vi "纳清pH电极校准.vi"() -> ()   [LabVIEW 2016, in "斯坦道多参数.lvlib"]
uses:
  <vilib>/Utility/miscctls.llb/LVPointTypeDef.ctl
  <vilib>/Analysis/NI_AALBase.lvlib
  <vilib>/ptbypt/NI_PtbyPt.lvlib
panel:
  out "第二点信号值":dbl
  out "第一点信号值":dbl
  out "报警信息":string
  out "通讯状态":string
  out "第二点校准值":dbl
  out "第一点校准值":dbl
  in  "校准停止":bool
  in  "校准启动":bool
  in  "校准模式":enum16{"两点校准", "单点校准"}(ring)
  out "最小值":sgl format="%#.2f"
  out "最大值":sgl format="%#.2f"
  out "波形图表":dbl(graph) caption="历史曲线"
  out "mean":dbl caption="均值" format="%#.2f"
  out "standard deviation":dbl caption="标准差" format="%#.2f"
  out "变异系数":dbl format="%#.6f"
  out "测量值":sgl format="%#.2f"
  out "提示":string
  out "标液2":sgl
  out "标液1":sgl
  out "原始光强数值":sgl caption="信号值" format="%#.6f"
  out "温度":dbl format="%#.2f"
  # "pH电极设定"
  # "℃"
  # "mV"
  # "请选择校准模式:"
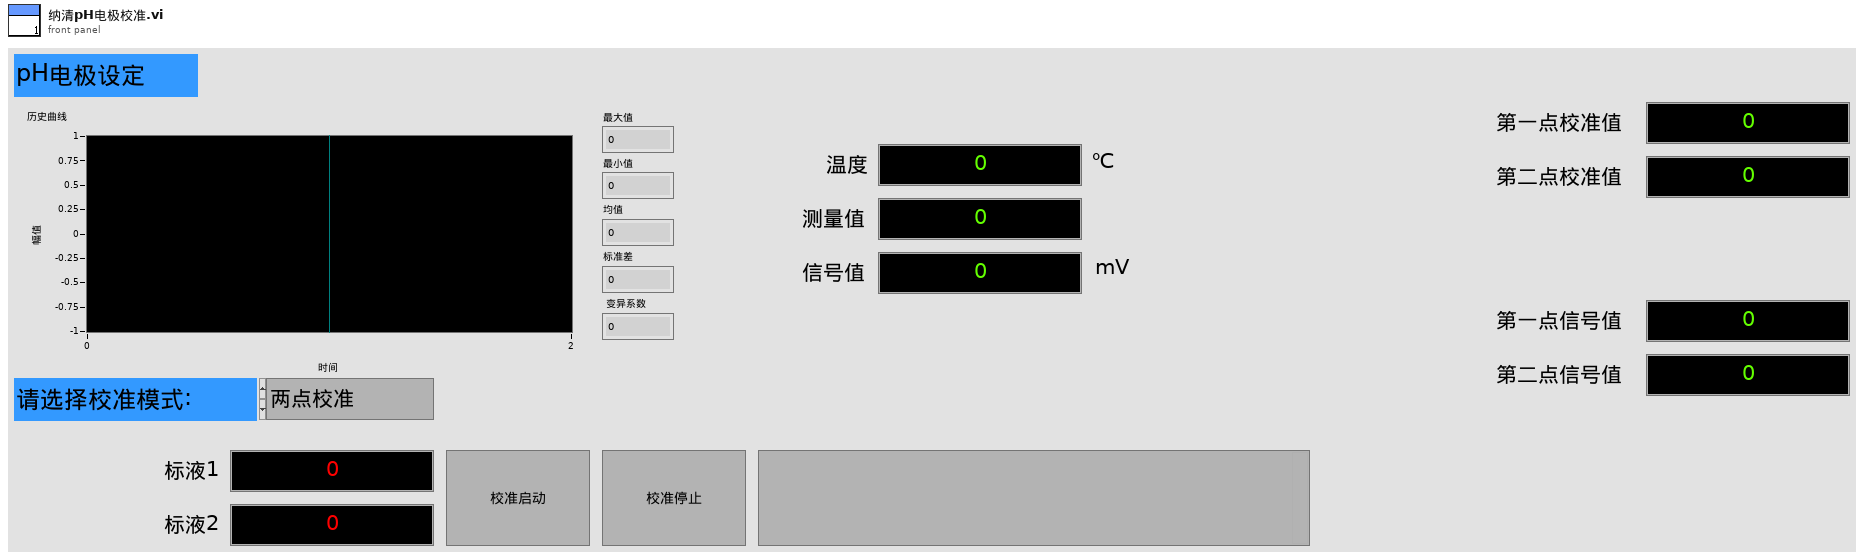
[diagram p1: front panel]
types:
  T1 = typedef "LVPointTypeDef.ctl" = cluster{"Horizontal":i16, "Vertical":i16}
  T2 = cluster{"报警码":u16, "pH数值":sgl, "0X0003_NC":sgl, "温度数据":sgl, "pH原始信号 mv":sgl, "0X0009_NC":string, "产品名称":string, "序列号":string, "硬件版本":string, "软件版本":string, "通讯地址":u16, "波特率":u16, "设备类型":u16, "0X0026_NC":string, "第一点原始数据":sgl, "第一点校准数据":sgl, "第二点原始数据":sgl, "第二点校准数据":sgl, "探头校准命令":u16, "温度校准参数":sgl, "温度校准命令":u16}
  T3 = enum8{"Enabled", "Disabled", "Disabled and Grayed Out"}
  T4 = cluster{"ph":bool, "DO":bool, "Cond":bool, "Turb":bool, "叶绿素a":bool, "藻密度":bool, "ORP":bool}
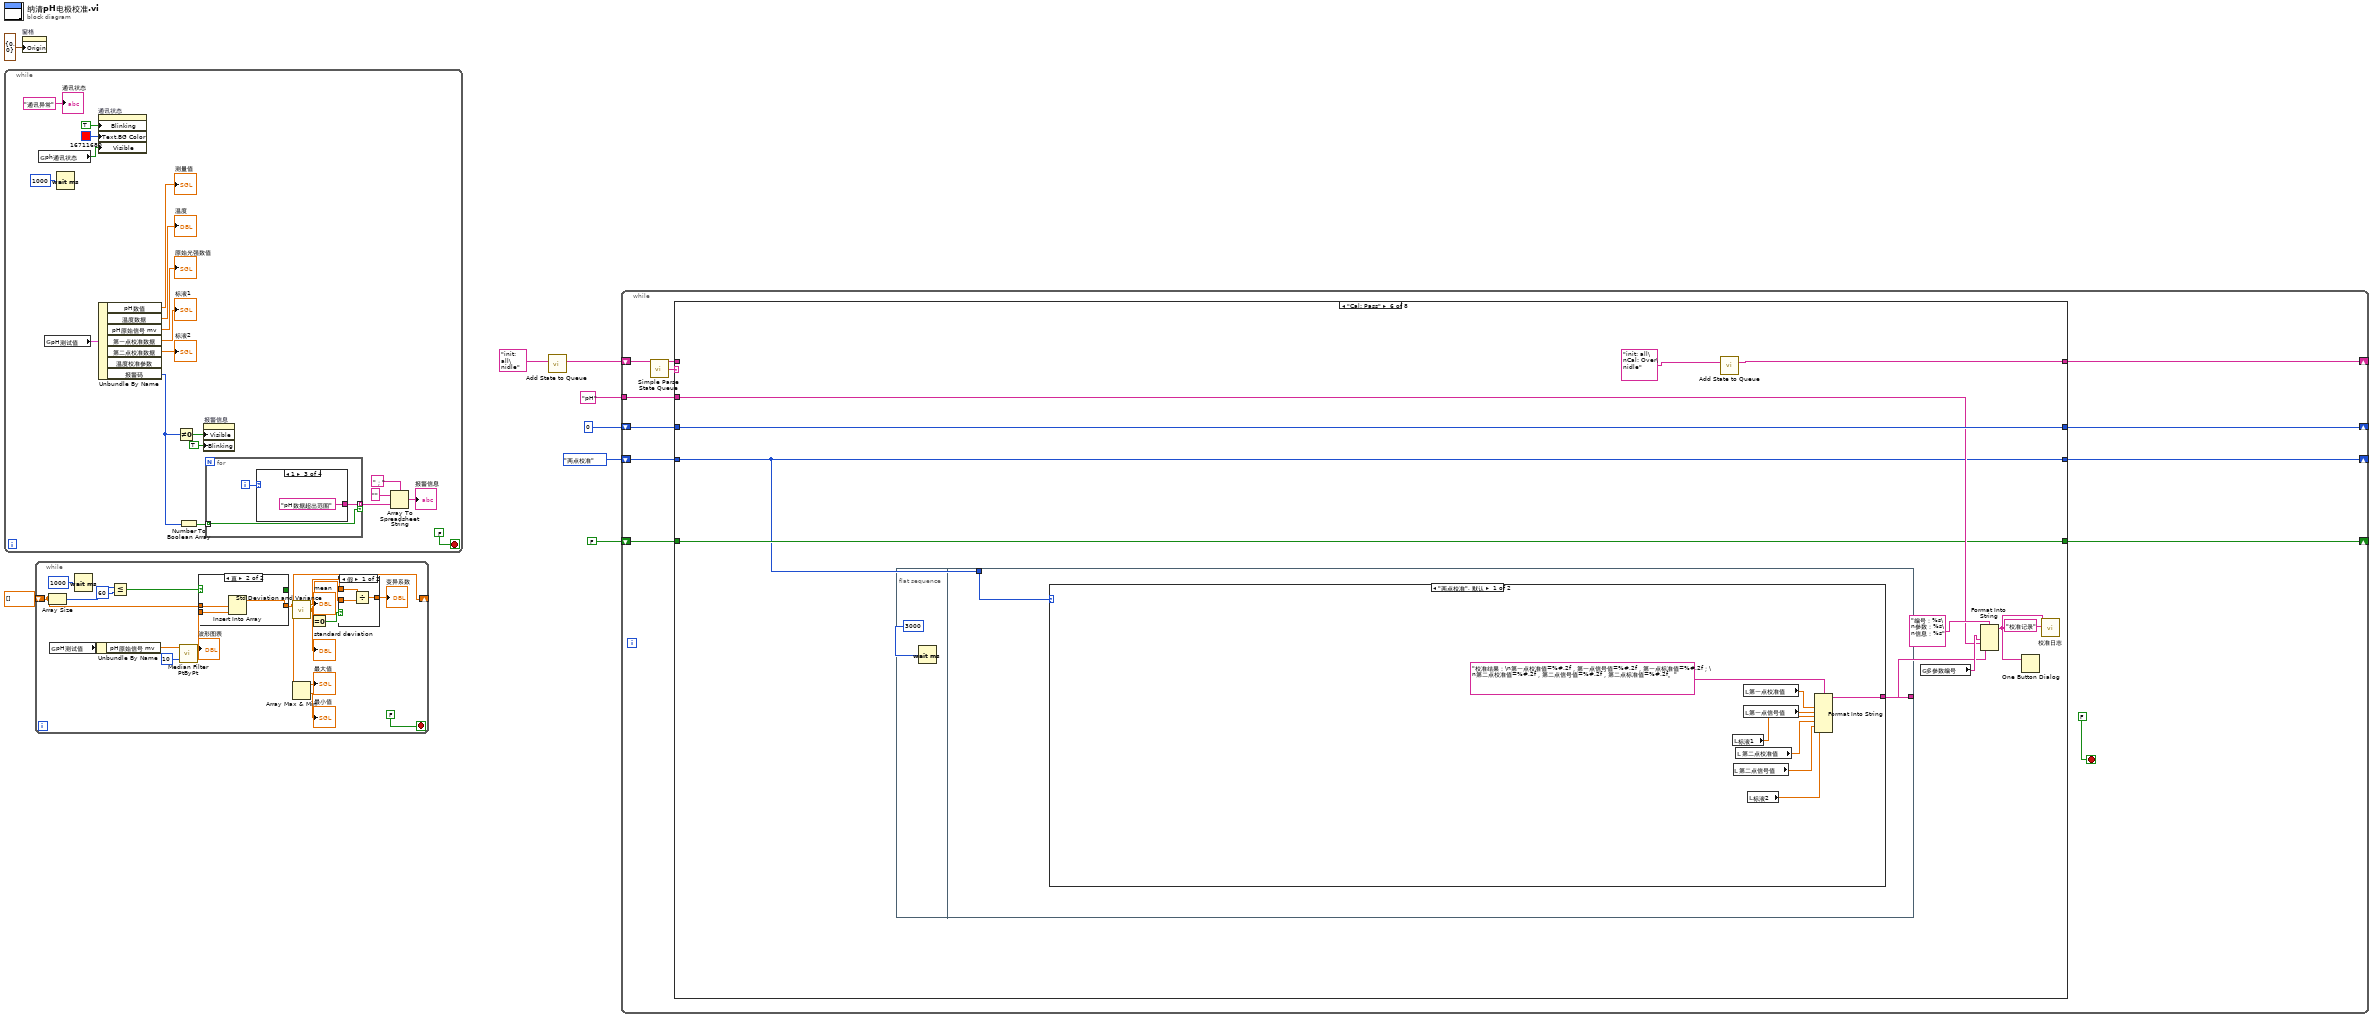
[diagram p0: block diagram]
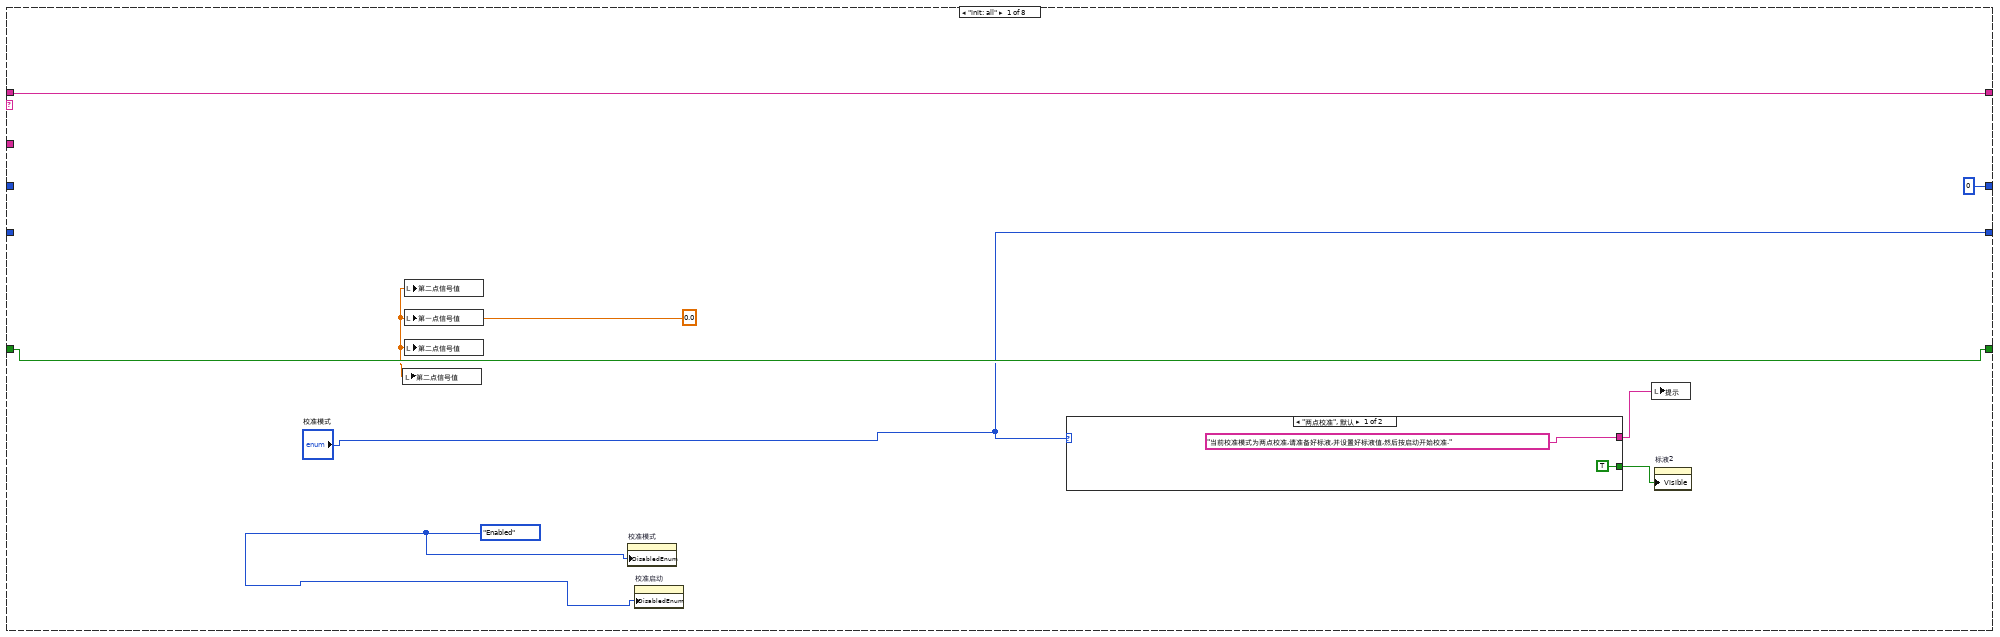
[diagram p2: hidden frame]
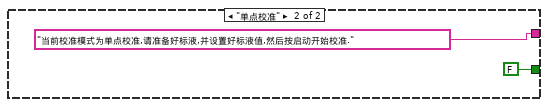
[diagram p3: hidden frame]
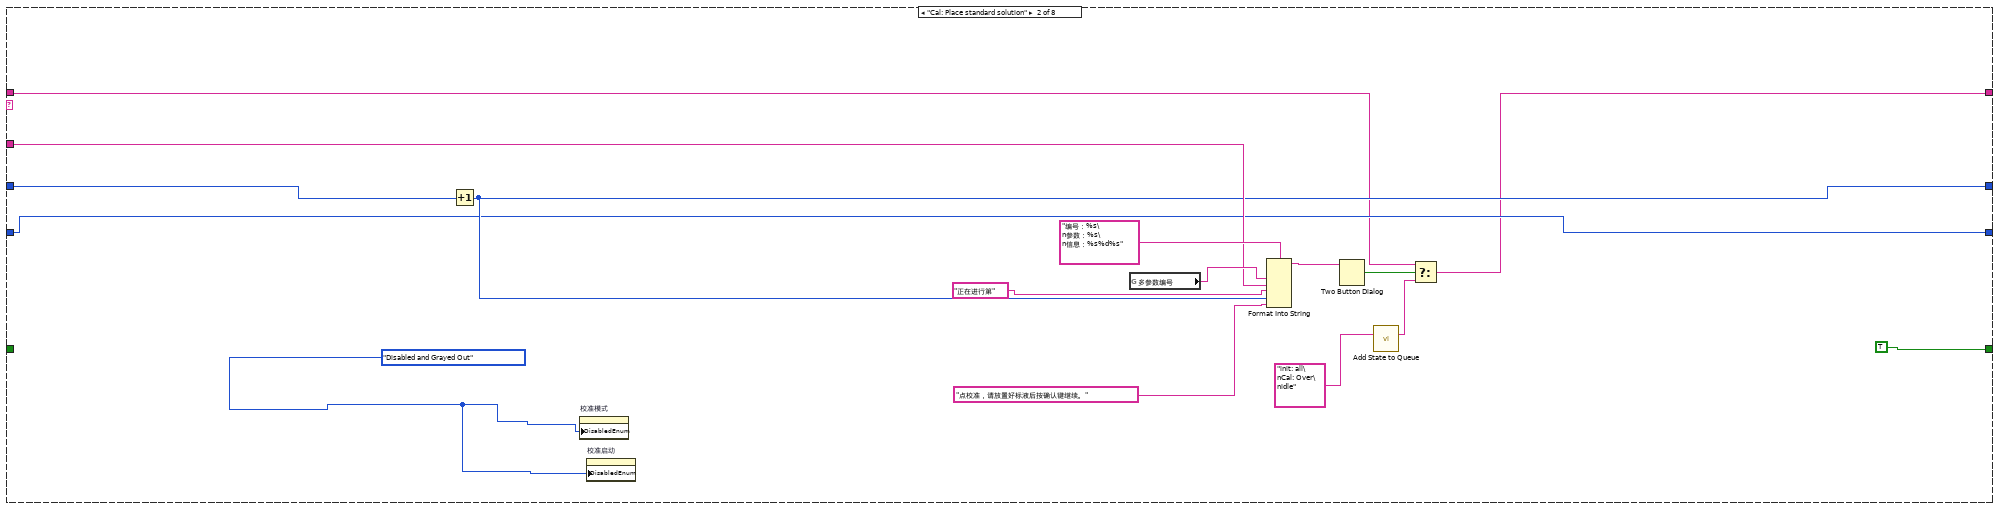
[diagram p4: hidden frame]
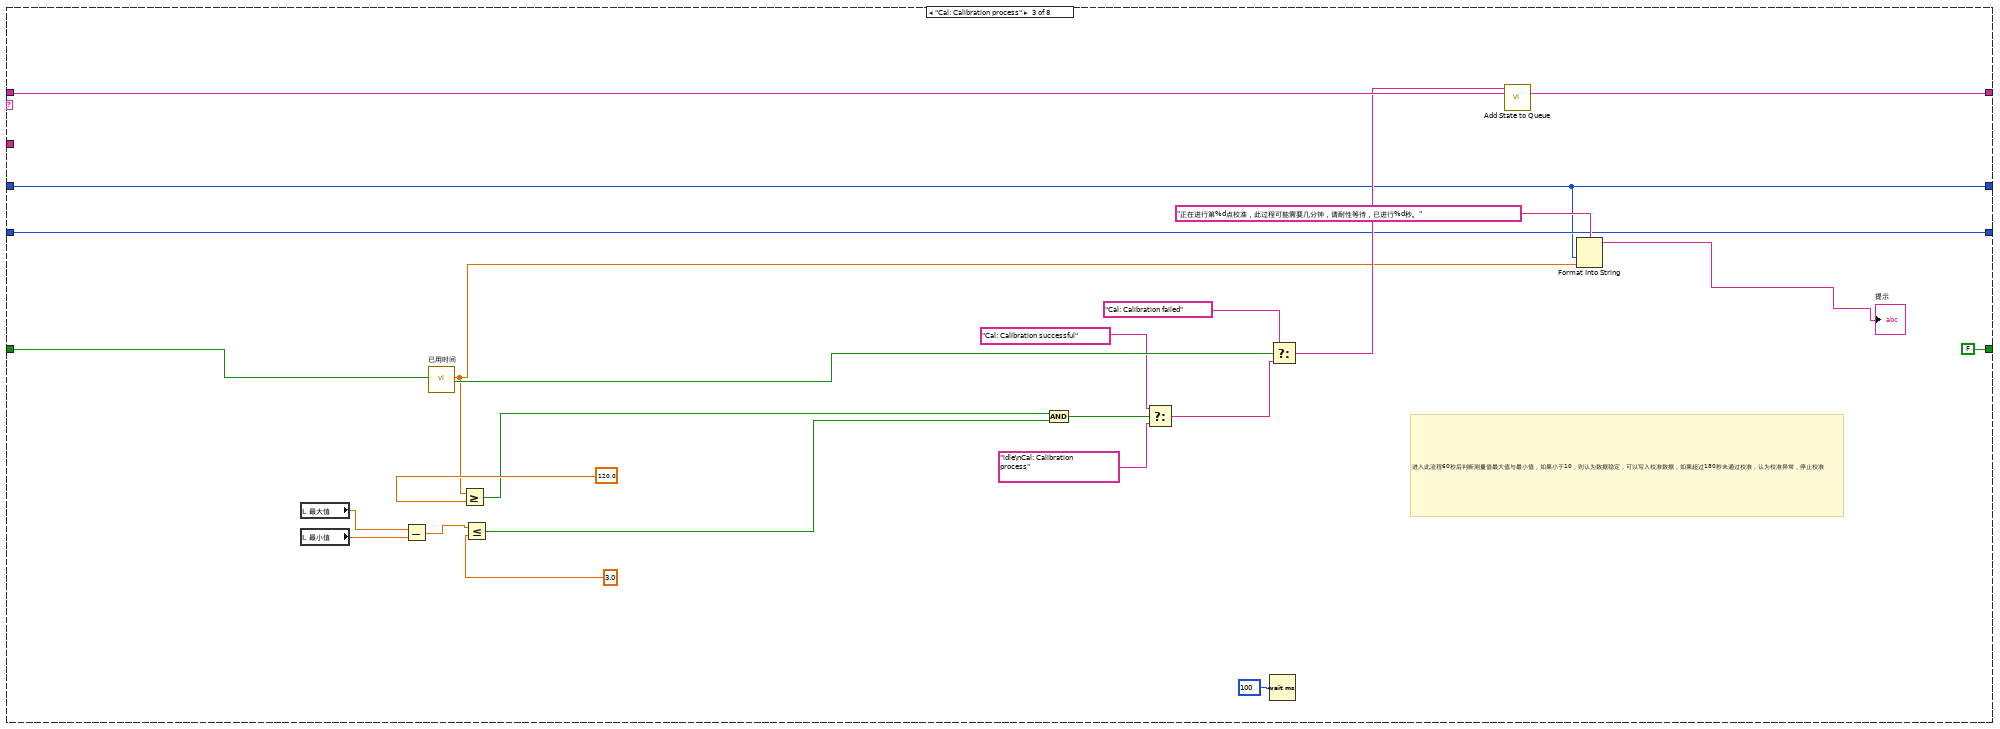
[diagram p5: hidden frame]
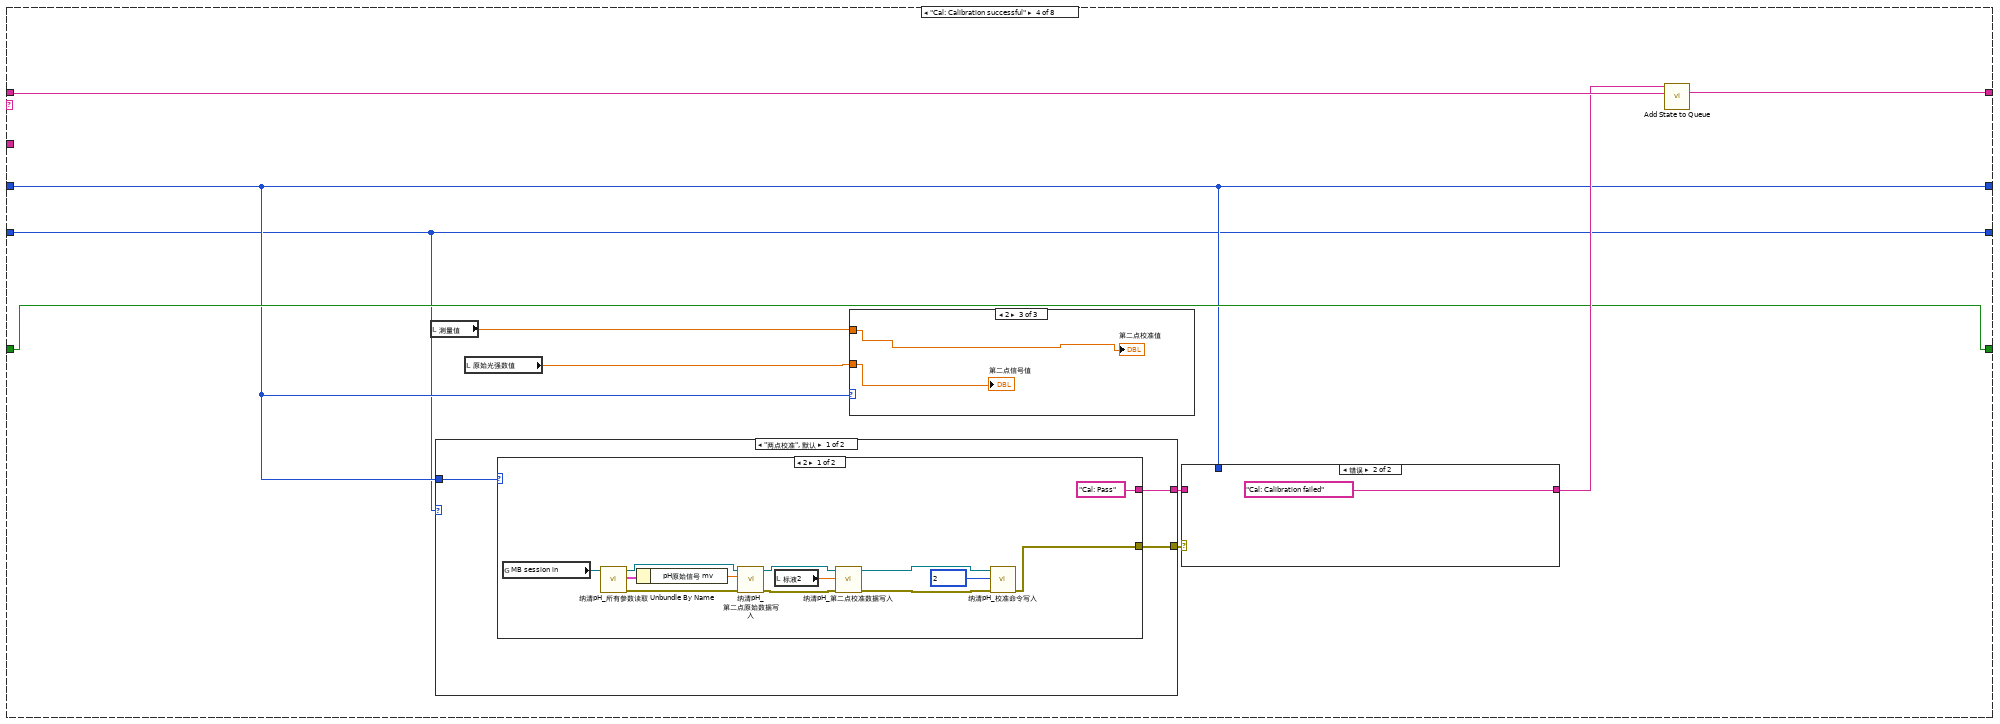
[diagram p6: hidden frame]
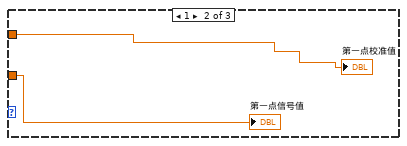
[diagram p8: hidden frame]
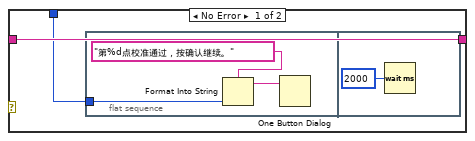
[diagram p9: hidden frame]
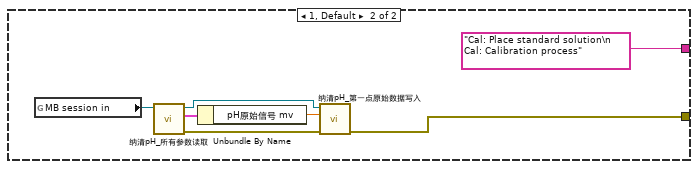
[diagram p10: hidden frame]
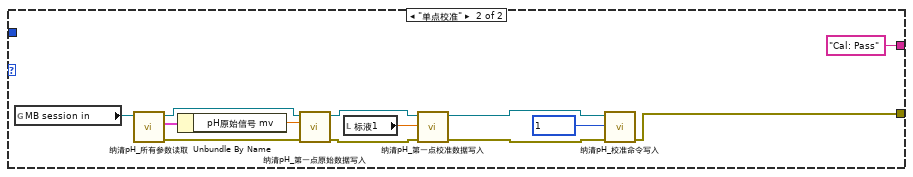
[diagram p11: hidden frame]
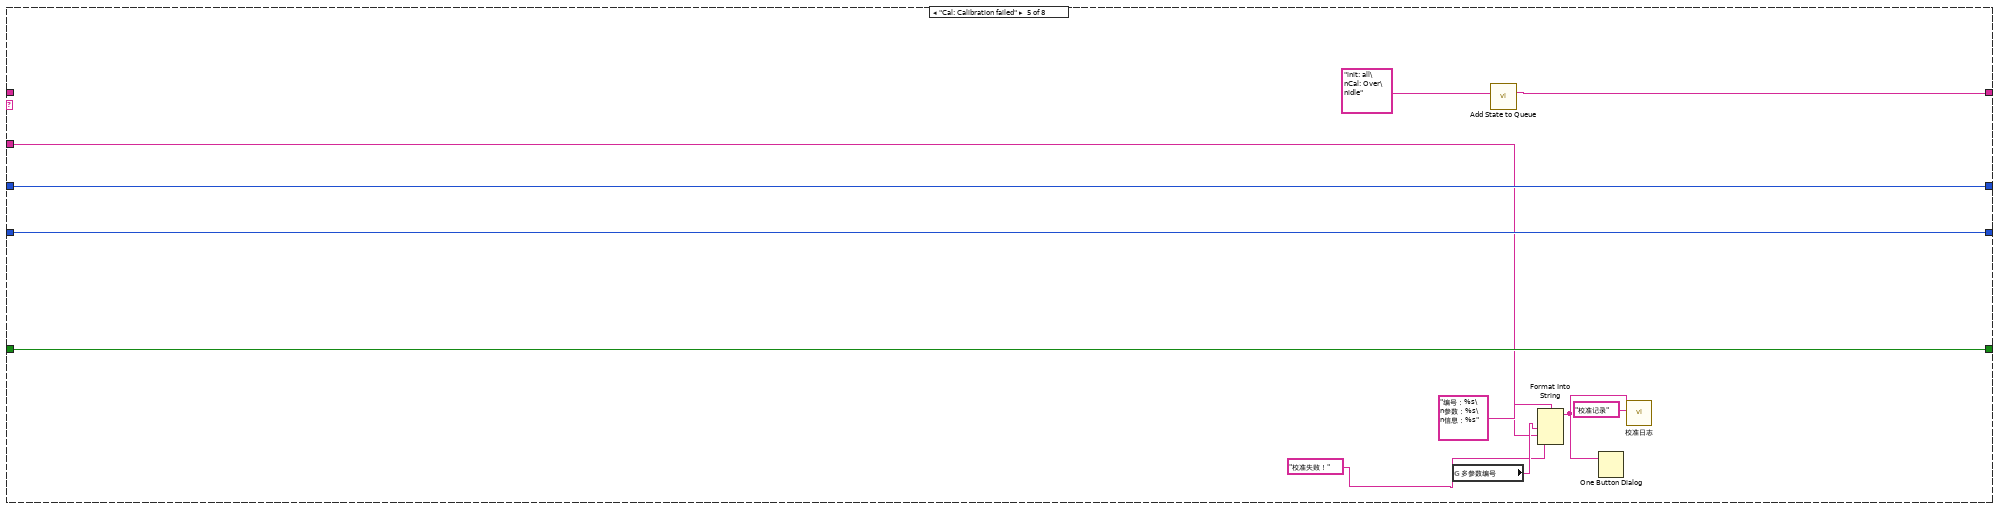
[diagram p12: hidden frame]
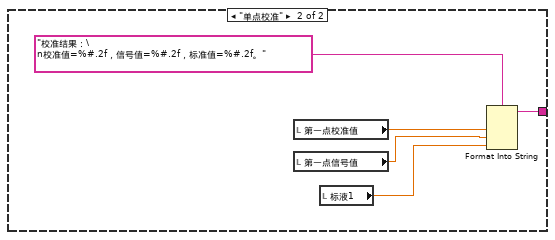
[diagram p13: hidden frame]
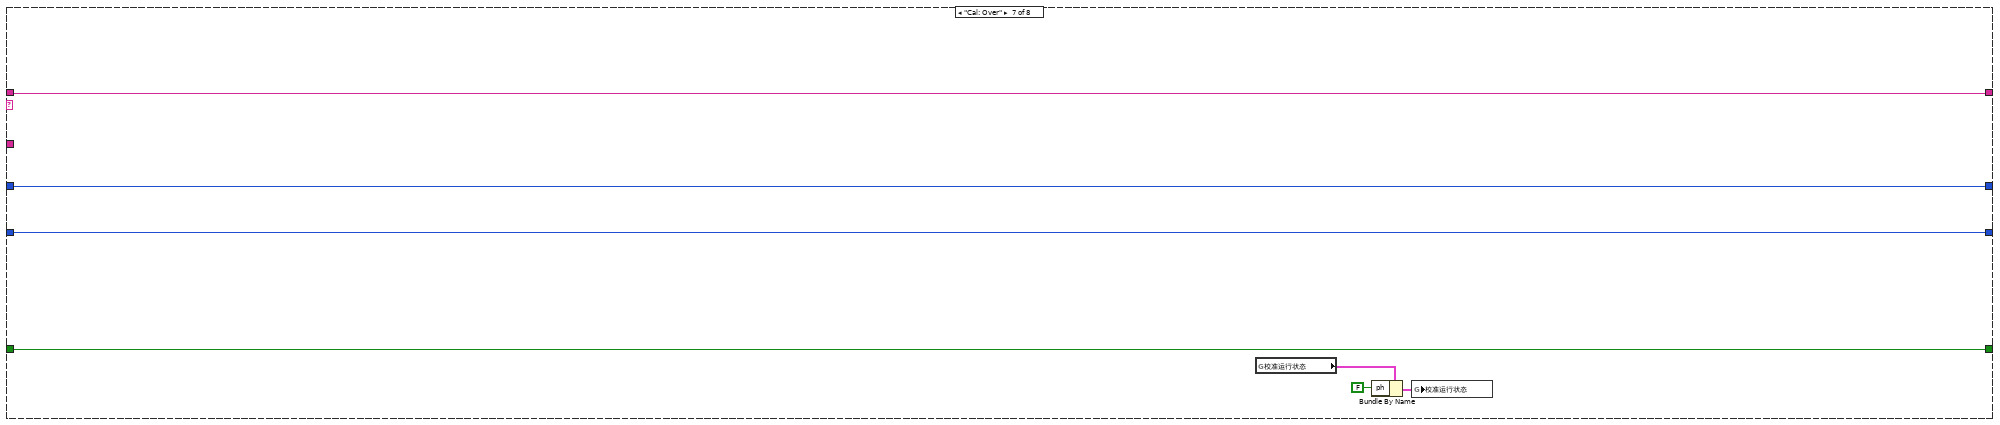
[diagram p14: hidden frame]
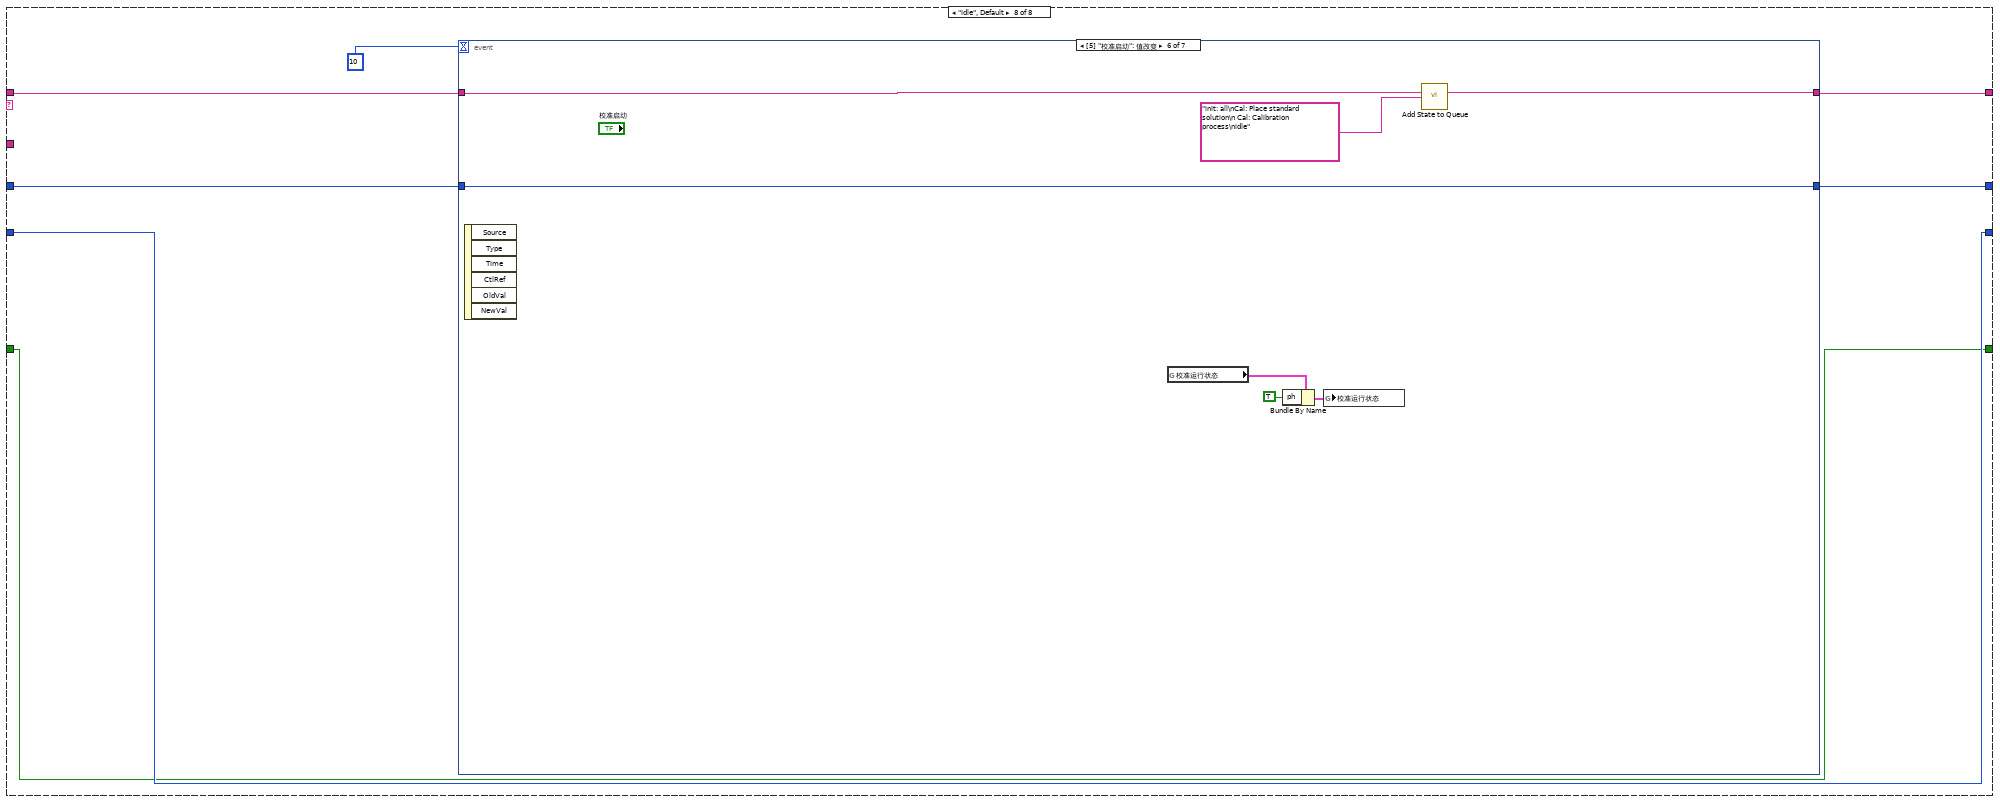
[diagram p15: hidden frame]
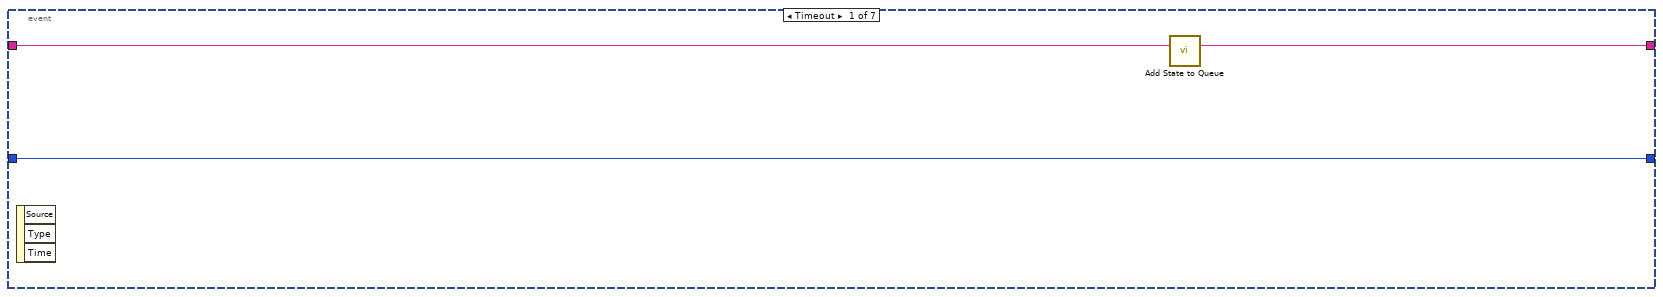
[diagram p16: hidden frame]
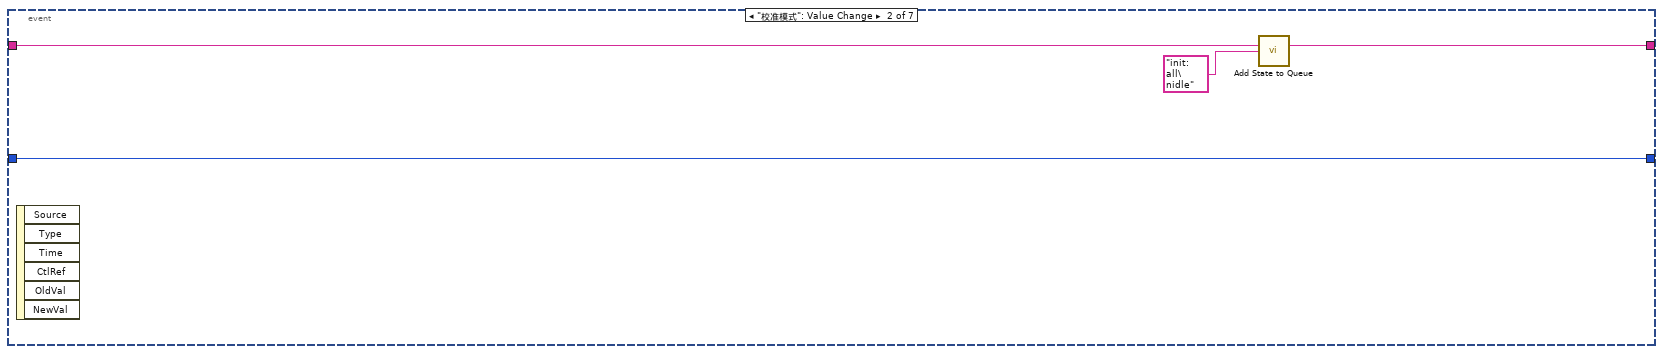
[diagram p17: hidden frame]
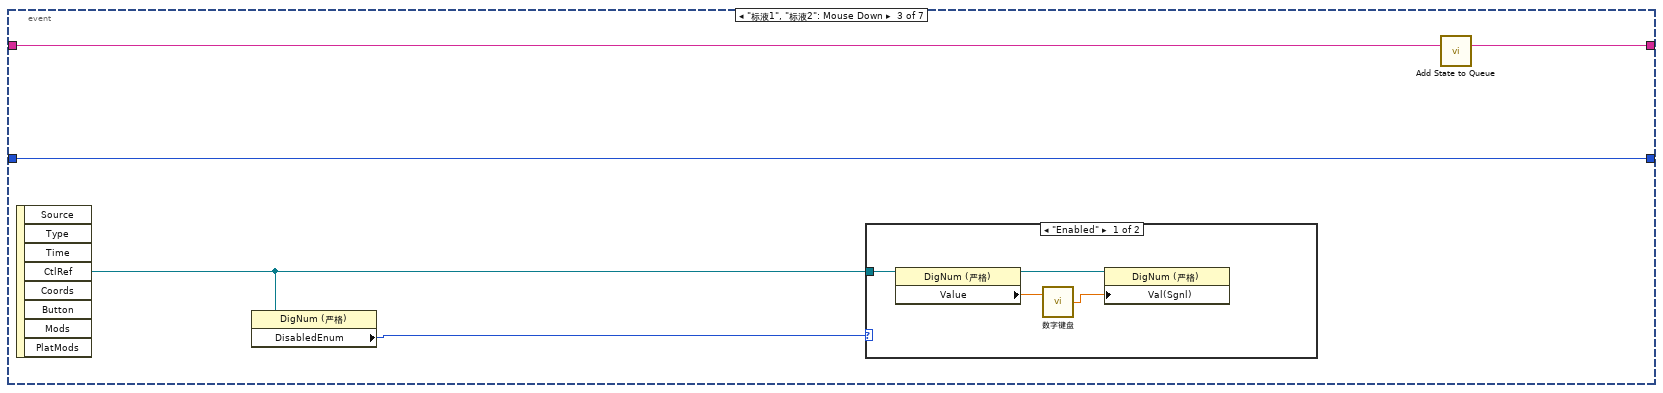
[diagram p18: hidden frame]
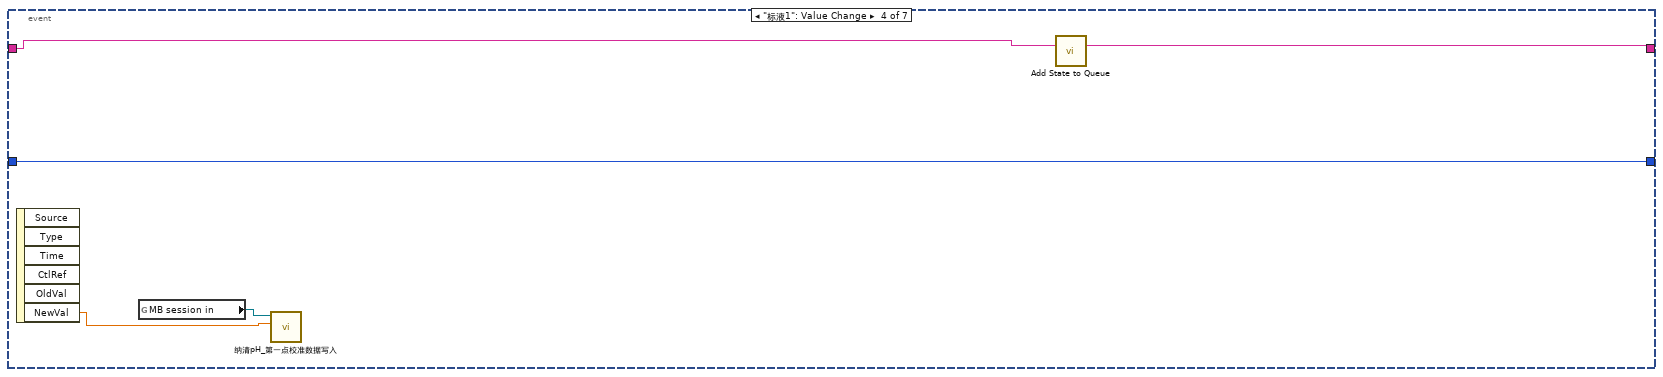
[diagram p20: hidden frame]
diagram:
  n1 = while {
    stop <- FALSE stop-if-true
    n2 = global read "多参数全局变量.vi" "ph通讯状态"() -> (w17:bool)
    n3 = global read "纳清过程全局变量.vi" "pH测试值"() -> (w26:T2)
    n4 = Wait (ms)(milliseconds to wait=u32 1000 ("等待时间（毫秒）")) -> ()  [unwired: 1 out]
    n5 = property on="通讯状态" class="Str"("Blinking"=TRUE ("闪烁"), "Text.BG Color"=u32 16711680, "Visible"=w17) -> ()  [unwired: 2 in, 2 out]
    n6 = Unbundle By Name(w26) -> ("pH数值"=→"测量值":sgl, "温度数据"=→"温度":sgl, "pH原始信号 mv"=→"原始光强数值":sgl, "第一点校准数据"=→"标液1":sgl, "第二点校准数据"=→"标液2":sgl, "报警码"=w11:u16)  [unwired: 1 out]
    n7 = Not Equal To 0?(x=w11) -> (x != 0?=w10:bool)
    n8 = Number To Boolean Array(number=w11) -> (Boolean array=w16:bool[])
    n9 = property on="报警信息" class="Str"("Visible"=w10, "Blinking"=TRUE ("闪烁")) -> ()  [unwired: 2 in, 2 out]
    n10 = for {
      tunnel: w16 -> [w29] mode=indexing
      tunnel: [w30] -> w15 mode=indexing if=w29
      i -> [w31]
      n11 = case shown="1" w31 {
        tunnel: [_ "温度超出范围" "pH数据超出范围" "温度传感器故障"] -> w30
        frame Default {
        }
        frame 0 {
        }
        frame 1 {
        }
        frame 8 {
        }
      }
    }
    n12 = Array To Spreadsheet String(delimiter (Tab)="；" ("分隔符(Tab)"), array=w15, 3:"" ("格式字符串")) -> (spreadsheet string=→"报警信息":string)
    "通讯状态" <- "通讯异常" ("当前串口")
  }
  n13 = property on="窗格" class="Pane"("Origin"=T1 {"Horizontal"=0, "Vertical"=0} ("原点")) -> ()  [unwired: 2 in, 2 out]
  n14 = while {
    shift-right: [w41] -> _
    shift-left: sgl[] [] -> [w47]
    stop <- FALSE stop-if-true
    n15 = Array Size(array=w47) -> (size(s)=w49:i32)
    n16 = global read "纳清过程全局变量.vi" "pH测试值"() -> (w38:T2)
    n17 = Wait (ms)(milliseconds to wait=u32 1000 ("等待时间（毫秒）")) -> ()  [unwired: 1 out]
    n18 = Unbundle By Name(w38) -> ("pH原始信号 mv"=w36:sgl)
    n19 = Less Or Equal?(x=w49, y=60) -> (x <= y?=w48:bool)
    n20 = call <vilib>:"Median Filter PtByPt.vi"("rank"=10, "x"=w36) -> ("Filtered x"=w35:dbl)  [unwired: 2 in, 1 out]
    "波形图表" <- w35
    n21 = case shown="真" w48 {
      tunnel: w47 -> [w60 w63]
      tunnel: w35 -> [w58 w62]
      tunnel: [w56 w61] -> w41
      tunnel: [TRUE _] -> _
      frame False {
        n22 = Replace Array Subset(array=w60, new element=w58) -> (w59:sgl[])  [unwired: 1 in]
        n23 = Rotate 1D Array(1:w59, 2:-1 ("n")) -> (0:w56:sgl[])
      }
      frame True {
        n24 = Insert Into Array(array=w63, new element=w62) -> (w61:sgl[])  [unwired: 1 in]
      }
    }
    n25 = call <vilib>:"Std Deviation and Variance.vi"("X"=w41) -> ("mean"=w45:dbl, "standard deviation"=w44:dbl)  [unwired: 1 in, 1 out]
    "mean" <- w45
    "standard deviation" <- w44
    n26 = Array Max & Min(array=w41) -> (max value=→"最大值":sgl, min value=→"最小值":sgl)  [unwired: 2 out]
    n27 = Equal To 0?(x=w45) -> (x = 0?=w46:bool)
    n28 = case shown="假" w46 {
      tunnel: w44 -> [w54 _]
      tunnel: [w53 _] -> w43
      tunnel: w45 -> [w52 _]
      frame False {
        n29 = Divide(x=w54, y=w52) -> (x/y=w53:dbl)
      }
      frame True {
      }
    }
    "变异系数" <- w43
  }
  n30 = call "Add State to Queue.vi"("State(s) In (\"\")"="init: all\nidle" ("State(s) In (\"\")")) -> ("States Out"=w5:string)  [unwired: 14 in]
  n31 = while {
    shift-right: [w71] -> _
    shift-left: w5 -> [w75]
    shift-right: [w68] -> _
    shift-left: 0 -> [w70]
    tunnel: "pH" ("State(s) In (\"\")") -> [w69]
    shift-right: [w66] -> _
    shift-left: enum16{"两点校准", "单点校准"}."两点校准" ("校准模式") -> [w67]
    shift-right: [w64] -> _
    shift-left: FALSE -> [w65]
    stop <- FALSE stop-if-true
    n32 = call "Simple Parse State Queue.vi"("State Queue"=w75) -> ("Remain States"=w72:string, "Next State"=w73:string)  [unwired: 13 in]
    n33 = case shown="\"Cal: Pass\"" w73 {
      tunnel: w72 -> [w83 w91 w122 w135 _ _ w229 w236]
      tunnel: [w83 w90 w121 w134 w192 w197 w229 w235] -> w71
      tunnel: w70 -> [_ w99 w106 w129 w195 w206 w228 w233]
      tunnel: w69 -> [_ w100 _ _ w186 w202 _ _]
      tunnel: [0 w97 w106 w129 w195 w206 w228 w234] -> w68
      tunnel: w67 -> [_ w96 w107 w128 w194 w198 w227 w232]
      tunnel: ["校准模式" w96 w107 w128 w194 w198 w227 w232] -> w66
      tunnel: w65 -> [w80 _ w109 w130 w193 w201 w226 w230]
      tunnel: [w80 TRUE FALSE w130 w193 w201 w226 w230] -> w64
      frame "init: all" {
        w78 = T3."Enabled" ("禁用")
        w79 = 0.0 ("第一点校准值")
        n34 = local write "第二点信号值"(w79) -> ()
        n35 = local write "第二点信号值"(w79) -> ()
        n36 = local write "第一点信号值"(w79) -> ()
        n37 = local write "第二点信号值"(w79) -> ()
        n38 = property on="校准模式" class="Enum (严格)"("DisabledEnum"=w78) -> ()  [unwired: 2 in, 2 out]
        n39 = property on="校准启动" class="Bool"("DisabledEnum"=w78) -> ()  [unwired: 2 in, 2 out]
        n40 = case shown="\"两点校准\", 默认" "校准模式" {
          tunnel: ["当前校准模式为两点校准,请准备好标液,并设置好标液值,然后按启动开始校准." ("提示") "当前校准模式为单点校准,请准备好标液,并设置好标液值,然后按启动开始校准." ("提示")] -> w82
          tunnel: [TRUE ("可见") FALSE ("可见")] -> w76
          frame "两点校准", Default {
          }
          frame "单点校准" {
          }
        }
        n41 = local write "提示"(w82) -> ()
        n42 = property on="标液2" class="DigNum (严格)"("Visible"=w76) -> ()  [unwired: 2 in, 2 out]
      }
      frame "Cal: Place standard solution" {
        w89 = T3."Disabled and Grayed Out" ("禁用")
        n43 = Increment(x=w99) -> (x+1=w97:i32)
        n44 = property on="校准模式" class="Enum (严格)"("DisabledEnum"=w89) -> ()  [unwired: 2 in, 2 out]
        n45 = property on="校准启动" class="Bool"("DisabledEnum"=w89) -> ()  [unwired: 2 in, 2 out]
        n46 = global read "多参数全局变量.vi" "多参数编号"() -> (w102:string)
        n47 = Format Into String(format string="编号：%s\n参数：%s\n信息：%s%d%s" ("格式字符串"), w102, w100, "正在进行第" ("消息"), w97, "点校准，请放置好标液后按确认键继续。" ("消息")) -> (resulting string=w94:string)  [unwired: 2 in, 1 out]
        n48 = Two Button Dialog(message=w94) -> (T button?=w93:bool)  [unwired: 2 in]
        n49 = call "Add State to Queue.vi"("State(s) In (\"\")"="init: all\nCal: Over\nidle" ("State(s) In (\"\")")) -> ("States Out"=w92:string)  [unwired: 14 in]
        n50 = Select(t=w91, s=w93, f=w92) -> (s? t:f=w90:string)
      }
      frame "Cal: Calibration process" {
        # "进入此流程60秒后判断测量值最大值与最小值，如果小于10，则认为数据稳定，可以写入校准数据，如果超过180秒未通过校准，认为校准异常，停止校准"
        n51 = local read "最大值"() -> (w126:sgl)
        n52 = local read "最小值"() -> (w125:sgl)
        n53 = Subtract(x=w126, y=w125) -> (x-y=w127:sgl)
        n54 = call "已用时间"("Reset"=w109) -> ("Elapsed Time (s)"=w105:dbl, "Time has Elapsed"=w123:bool)  [unwired: 11 in, 6 out]
        n55 = Greater Or Equal?(x=w105, y=120.0) -> (x >= y?=w118:bool)
        n56 = Less Or Equal?(x=w127, y=3.0) -> (x <= y?=w114:bool)
        n57 = And(x=w118, y=w114) -> (x .and. y?=w115:bool)
        n58 = Select(t="Cal: Calibration successful" ("State(s) In (\"\")"), s=w115, f="idle\nCal: Calibration process" ("State(s) In (\"\")")) -> (s? t:f=w113:string)
        n59 = Wait (ms)(milliseconds to wait=u32 100 ("等待时间（毫秒）")) -> ()  [unwired: 1 out]
        n60 = Select(t="Cal: Calibration failed" ("State(s) In (\"\")"), s=w123, f=w113) -> (s? t:f=w112:string)
        n61 = call "Add State to Queue.vi"("State(s) In Front (\"\")"=w112, "State(s) In (\"\")"=w122) -> ("States Out"=w121:string)  [unwired: 13 in]
        n62 = Format Into String(format string="正在进行第%d点校准，此过程可能需要几分钟，请耐性等待，已进行%d秒。" ("格式字符串"), w106, w105) -> (resulting string=→"提示":string)  [unwired: 2 in, 1 out]
      }
      frame "Cal: Calibration successful" {
        n63 = local read "测量值"() -> (w131:sgl)
        n64 = case shown="\"两点校准\", 默认" w128 {
          tunnel: [w151 w172] -> w137
          tunnel: [w150 "Cal: Pass" ("State(s) In (\"\")")] -> w136
          tunnel: w129 -> [w149 _]
          frame "两点校准", Default {
            n65 = case shown="2" w149 {
              tunnel: [w152 w165] -> w151
              tunnel: ["Cal: Pass" ("State(s) In (\"\")") "Cal: Place standard solution\n Cal: Calibration process" ("State(s) In (\"\")")] -> w150
              frame 2 {
                n66 = global read "多参数全局变量.vi" "MB session in"() -> (w160:refnum<class "MB_Master.lvclass">)
                n67 = call "纳清pH_所有参数读取.vi"("MB session in"=w160) -> ("error out"=w162:errorcluster, "输出值"=w159:T2, "MB session out"=w161:refnum<class "MB_Master.lvclass">)  [unwired: 8 in]
                n68 = Unbundle By Name(w159) -> ("pH原始信号 mv"=w158:sgl)
                n69 = call "纳清pH_第二点原始数据写入.vi"("error in (no error)"=w162, "数值"=w158, "MB session in"=w161) -> ("error out"=w157:errorcluster, "MB session out"=w156:refnum<class "MB_Master.lvclass">)  [unwired: 7 in]
                n70 = local read "标液2"() -> (w153:sgl)
                n71 = call "纳清pH_第二点校准数据写入.vi"("error in (no error)"=w157, "数值"=w153, "MB session in"=w156) -> ("error out"=w155:errorcluster, "MB session out"=w154:refnum<class "MB_Master.lvclass">)  [unwired: 7 in]
                n72 = call "纳清pH_校准命令写入.vi"("error in (no error)"=w155, "数值"=u16 2 ("starting address"), "MB session in"=w154) -> ("error out"=w152:errorcluster)  [unwired: 7 in, 1 out]
              }
              frame 1, Default {
                n73 = global read "多参数全局变量.vi" "MB session in"() -> (w168:refnum<class "MB_Master.lvclass">)
                n74 = call "纳清pH_所有参数读取.vi"("MB session in"=w168) -> ("error out"=w170:errorcluster, "输出值"=w167:T2, "MB session out"=w169:refnum<class "MB_Master.lvclass">)  [unwired: 8 in]
                n75 = Unbundle By Name(w167) -> ("pH原始信号 mv"=w166:sgl)
                n76 = call "纳清pH_第一点原始数据写入.vi"("error in (no error)"=w170, "数值"=w166, "MB session in"=w169) -> ("error out"=w165:errorcluster)  [unwired: 7 in, 1 out]
              }
            }
          }
          frame "单点校准" {
            n77 = global read "多参数全局变量.vi" "MB session in"() -> (w180:refnum<class "MB_Master.lvclass">)
            n78 = call "纳清pH_所有参数读取.vi"("MB session in"=w180) -> ("error out"=w182:errorcluster, "输出值"=w179:T2, "MB session out"=w181:refnum<class "MB_Master.lvclass">)  [unwired: 8 in]
            n79 = Unbundle By Name(w179) -> ("pH原始信号 mv"=w178:sgl)
            n80 = call "纳清pH_第一点原始数据写入.vi"("error in (no error)"=w182, "数值"=w178, "MB session in"=w181) -> ("error out"=w177:errorcluster, "MB session out"=w176:refnum<class "MB_Master.lvclass">)  [unwired: 7 in]
            n81 = local read "标液1"() -> (w173:sgl)
            n82 = call "纳清pH_第一点校准数据写入.vi"("error in (no error)"=w177, "数值"=w173, "MB session in"=w176) -> ("error out"=w175:errorcluster, "MB session out"=w174:refnum<class "MB_Master.lvclass">)  [unwired: 7 in]
            n83 = call "纳清pH_校准命令写入.vi"("error in (no error)"=w175, "数值"=u16 1 ("starting address"), "MB session in"=w174) -> ("error out"=w172:errorcluster)  [unwired: 7 in, 1 out]
          }
        }
        n84 = local read "原始光强数值"() -> (w132:sgl)
        n85 = case shown="2" w129 {
          tunnel: w132 -> [_ w139 w141]
          tunnel: w131 -> [_ w138 w140]
          frame 0, Default {
          }
          frame 1 {
            "第一点信号值" <- w139
            "第一点校准值" <- w138
          }
          frame 2 {
            "第二点信号值" <- w141
            "第二点校准值" <- w140
          }
        }
        n86 = case shown="错误" w137 {
          tunnel: w136 -> [w143 _]
          tunnel: [w143 "Cal: Calibration failed" ("State(s) In (\"\")")] -> w133
          tunnel: w129 -> [w142 _]
          frame No Error {
            n87 = flat-sequence {
              tunnel: w142 -> [w144]
              frame #0 {
                n88 = Format Into String(format string="第%d点校准通过，按确认继续。" ("格式字符串"), w144) -> (resulting string=w146:string)  [unwired: 2 in, 1 out]
                n89 = One Button Dialog(message=w146) -> ()  [unwired: 1 in, 1 out]
              }
              frame #1 {
                n90 = Wait (ms)(milliseconds to wait=u32 2000 ("等待时间（毫秒）")) -> ()  [unwired: 1 out]
              }
            }
          }
          frame Error {
          }
        }
        n91 = call "Add State to Queue.vi"("State(s) In Front (\"\")"=w133, "State(s) In (\"\")"=w135) -> ("States Out"=w134:string)  [unwired: 13 in]
      }
      frame "Cal: Calibration failed" {
        n92 = global read "多参数全局变量.vi" "多参数编号"() -> (w189:string)
        n93 = call "Add State to Queue.vi"("State(s) In (\"\")"="init: all\nCal: Over\nidle" ("State(s) In (\"\")")) -> ("States Out"=w192:string)  [unwired: 14 in]
        n94 = Format Into String(format string="编号：%s\n参数：%s\n信息：%s" ("格式字符串"), w189, w186, "校准失败！" ("消息")) -> (resulting string=w188:string)  [unwired: 2 in, 1 out]
        n95 = One Button Dialog(message=w188) -> ()  [unwired: 1 in, 1 out]
        n96 = call "校准日志.vi"("table"="校准记录", "日志信息"=w188) -> ()  [unwired: 9 in, 1 out]
      }
      frame "Cal: Pass" {
        n97 = flat-sequence {
          tunnel: [w209] -> w199
          tunnel: w198 -> [w208]
          frame #0 {
            n98 = Wait (ms)(milliseconds to wait=u32 3000 ("等待时间（毫秒）")) -> ()  [unwired: 1 out]
          }
          frame #1 {
            n99 = case shown="\"两点校准\", 默认" w208 {
              tunnel: [w217 w222] -> w209
              frame "两点校准", Default {
                n100 = local read "标液1"() -> (w213:sgl)
                n101 = local read "第二点信号值"() -> (w211:dbl)
                n102 = local read "第二点校准值"() -> (w212:dbl)
                n103 = local read "第一点校准值"() -> (w215:dbl)
                n104 = local read "第一点信号值"() -> (w216:dbl)
                n105 = local read "标液2"() -> (w210:sgl)
                n106 = Format Into String(format string="校准结果：\n第一点校准值=%#.2f，第一点信号值=%#.2f，第一点标准值=%#.2f；\n第二点校准值=%#.2f，第二点信号值=%#.2f，第二点标准值=%#.2f。" ("提示"), w215, w216, w213, w212, w211, w210) -> (resulting string=w217:string)  [unwired: 2 in, 1 out]
              }
              frame "单点校准" {
                n107 = local read "第一点校准值"() -> (w221:dbl)
                n108 = local read "第一点信号值"() -> (w219:dbl)
                n109 = local read "标液1"() -> (w218:sgl)
                n110 = Format Into String(format string="校准结果：\n校准值=%#.2f，信号值=%#.2f，标准值=%#.2f。" ("提示"), w221, w219, w218) -> (resulting string=w222:string)  [unwired: 2 in, 1 out]
              }
            }
          }
        }
        n111 = call "Add State to Queue.vi"("State(s) In (\"\")"="init: all\nCal: Over\nidle" ("State(s) In (\"\")")) -> ("States Out"=w197:string)  [unwired: 14 in]
        n112 = global read "多参数全局变量.vi" "多参数编号"() -> (w203:string)
        n113 = Format Into String(format string="编号：%s\n参数：%s\n信息：%s" ("格式字符串"), w203, w202, w199) -> (resulting string=w200:string)  [unwired: 2 in, 1 out]
        n114 = One Button Dialog(message=w200) -> ()  [unwired: 1 in, 1 out]
        n115 = call "校准日志.vi"("table"="校准记录", "日志信息"=w200) -> ()  [unwired: 9 in, 1 out]
      }
      frame "Cal: Over" {
        n116 = global read "多参数全局变量.vi" "校准运行状态"() -> (w224:T4)
        n117 = Bundle By Name(cluster=w224, "ph"=FALSE) -> (w225:T4)
        n118 = global write "多参数全局变量.vi" "校准运行状态"(w225) -> ()
      }
      frame "idle", Default {
        n119 = event shown="[5] \"校准启动\": 值改变" {
          selector: _ -> [_ _ _ _ _ _ _]
          dyn-events: _ -> [_ _ _ _ _ _ _]
          timeout: 10 -> [_ _ _ _ _ _ _]
          tunnel: w236 -> [w239 w243 w246 w253 w258 w269 _]
          tunnel: [w238 w242 w247 w257 w262 w268 w271] -> w235
          tunnel: [w237 w240 w248 w256 w261 w266 w272] -> w234
          tunnel: w233 -> [w237 w240 w248 w256 w261 w266 w272]
          event Timeout {
            n120 = event-data() -> ()  [unwired: 1 in, 3 out]
            n121 = call "Add State to Queue.vi"("State(s) In (\"\")"=w239) -> ("States Out"=w238:string)  [unwired: 14 in]
          }
          event "校准模式": Value Change {
            n122 = event-data() -> ()  [unwired: 1 in, 6 out]
            n123 = call "Add State to Queue.vi"("State(s) In (\"\")"=w243, "State(s) At Back (\"\")"="init: all\nidle" ("State(s) In (\"\")")) -> ("States Out"=w242:string)  [unwired: 13 in]
          }
          event "标液1", "标液2": Mouse Down {
            n124 = event-data() -> ("CtlRef"=w245:refnum<vi>)  [unwired: 1 in, 7 out]
            n125 = property class="DigNum (严格)"(reference=w245) -> ("DisabledEnum"=w244:T3)  [unwired: 1 in, 2 out]
            n126 = case shown="\"Enabled\"" w244 {
              tunnel: w245 -> [w252 _]
              frame "Enabled" {
                n127 = property class="DigNum (严格)"(reference=w252) -> (reference out=w249:refnum<vi>, "Value"=w250:sgl)  [unwired: 1 in, 1 out]
                n128 = call "数字键盘.vi"("OldNumber"=w250) -> ("NewNumber"=w251:dbl)  [unwired: 1 in]
                n129 = property class="DigNum (严格)"(reference=w249, "Val(Sgnl)"=w251) -> ()  [unwired: 1 in, 2 out]
              }
              frame "Disabled", Default {
              }
            }
            n130 = call "Add State to Queue.vi"("State(s) In (\"\")"=w246) -> ("States Out"=w247:string)  [unwired: 14 in]
          }
          event "标液1": Value Change {
            n131 = event-data() -> ("NewVal"=w254:sgl)  [unwired: 1 in, 5 out]
            n132 = global read "多参数全局变量.vi" "MB session in"() -> (w255:refnum<class "MB_Master.lvclass">)
            n133 = call "纳清pH_第一点校准数据写入.vi"("数值"=w254, "MB session in"=w255) -> ()  [unwired: 8 in, 2 out]
            n134 = call "Add State to Queue.vi"("State(s) In (\"\")"=w253) -> ("States Out"=w257:string)  [unwired: 14 in]
          }
          event "标液2": Value Change {
            n135 = event-data() -> ("NewVal"=w259:sgl)  [unwired: 1 in, 5 out]
            n136 = global read "多参数全局变量.vi" "MB session in"() -> (w260:refnum<class "MB_Master.lvclass">)
            n137 = call "纳清pH_第二点校准数据写入.vi"("数值"=w259, "MB session in"=w260) -> ()  [unwired: 8 in, 2 out]
            n138 = call "Add State to Queue.vi"("State(s) In (\"\")"=w258) -> ("States Out"=w262:string)  [unwired: 14 in]
          }
          event "校准启动": Value Change {
            n139 = event-data() -> ()  [unwired: 1 in, 6 out]
            n140 = global read "多参数全局变量.vi" "校准运行状态"() -> (w264:T4)
            n141 = Bundle By Name(cluster=w264, "ph"=TRUE) -> (w265:T4)
            n142 = global write "多参数全局变量.vi" "校准运行状态"(w265) -> ()
            n143 = call "Add State to Queue.vi"("State(s) In (\"\")"=w269, "State(s) At Back (\"\")"="init: all\nCal: Place standard solution\n Cal: Calibration process\nidle" ("State(s) In (\"\")")) -> ("States Out"=w268:string)  [unwired: 13 in]
          }
          event "校准停止": Value Change {
            n144 = event-data() -> ()  [unwired: 1 in, 6 out]
            n145 = call "Add State to Queue.vi"("State(s) In (\"\")"="init: all\nCal: Over\nidle" ("State(s) In (\"\")")) -> ("States Out"=w271:string)  [unwired: 14 in]
          }
        }
      }
    }
  }
